vi "Configure Measurement (Spectrum Emission Mask).vi"(0 "VISA resource name":refnum<visa-resource-name>, 1 "Channel Span (2E+7 Hz)":dbl=20000000.0, 2 "Enable Averaging (T: Enable)":bool=TRUE, 5 "Auto Resolution Bandwidth (T: Enable)":bool=TRUE, 7 "Resolution Bandwidth (30 Hz)":dbl=30.0, 9 "Center Frequency (1E+9 Hz)":dbl=1000000000.0, 11 "error in (no error)":errorcluster, 12 "Average Number (20)":dbl=20.0) -> (4 "VISA resource name out":refnum<visa-resource-name>, 15 "error out":errorcluster)   [LabVIEW 2022 SP3, in "Agilent N934X Series.lvlib"]
doc: "Sets the Spectrum Emission Mask measurement parameters.\n\nNote:\nThis VI is only applicable for N9321C, N9322C, N9323C, N9324C models"
uses:
  <instrlib>/Agilent N934X Series/Agilent N934X Series.lvlib
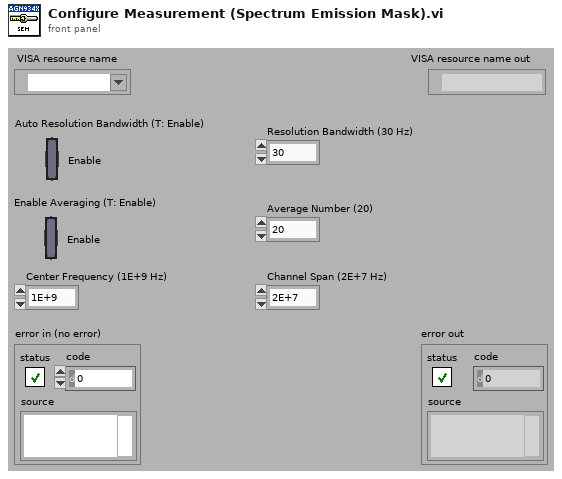
[diagram p1: front panel]
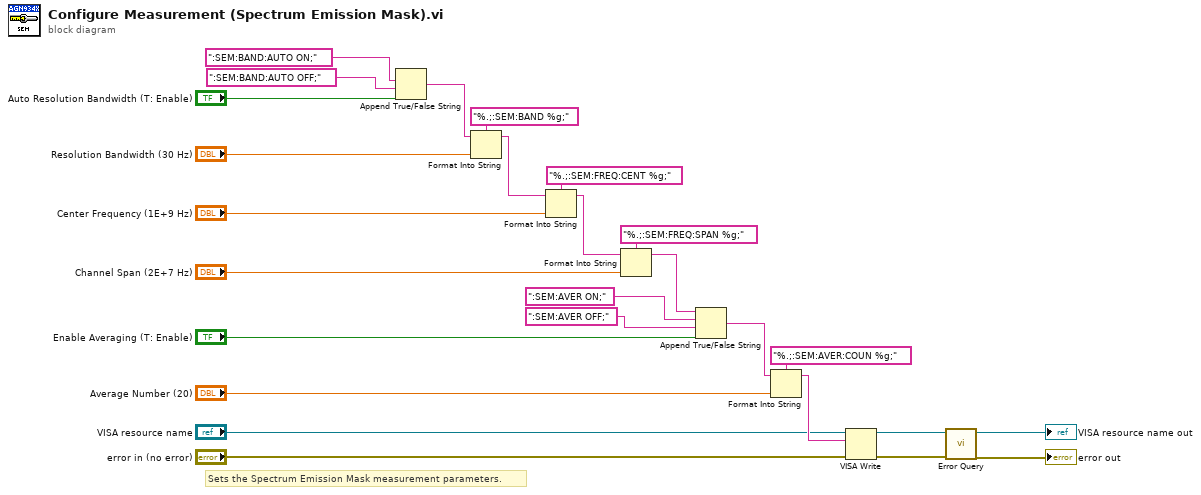
[diagram p0: block diagram]
diagram:
  # "Sets the Spectrum Emission Mask measurement parameters."
  n1 = Append True/False String(1:"Auto Resolution Bandwidth (T: Enable)", 2:":SEM:BAND:AUTO OFF;", 3:":SEM:BAND:AUTO ON;") -> (0:w23:string)  [unwired: 1 in]
  n2 = Format Into String(format string="%.;:SEM:BAND %g;", initial string=w23, "Resolution Bandwidth (30 Hz)") -> (resulting string=w20:string)  [unwired: 1 in, 1 out]
  n3 = Format Into String(format string="%.;:SEM:FREQ:CENT %g;", initial string=w20, "Center Frequency (1E+9 Hz)") -> (resulting string=w17:string)  [unwired: 1 in, 1 out]
  n4 = Format Into String(format string="%.;:SEM:FREQ:SPAN %g;", initial string=w17, "Channel Span (2E+7 Hz)") -> (resulting string=w14:string)  [unwired: 1 in, 1 out]
  n5 = Append True/False String(1:"Enable Averaging (T: Enable)", 2:":SEM:AVER OFF;", 3:":SEM:AVER ON;", 4:w14) -> (0:w10:string)
  n6 = Format Into String(format string="%.;:SEM:AVER:COUN %g;", initial string=w10, "Average Number (20)") -> (resulting string=w7:string)  [unwired: 1 in, 1 out]
  n7 = VISA Write(VISA resource name="VISA resource name", write buffer=w7, error in (no error)="error in (no error)") -> (VISA resource name out=w4:refnum<visa-resource-name>, error out=w3:errorcluster)  [unwired: 1 out]
  n8 = call <instrlib>:"Error Query.vi"("error in (no error)"=w3, "VISA resource name"=w4) -> ("error out"=→"error out":errorcluster, "VISA resource name out"=→"VISA resource name out":refnum<visa-resource-name>)  [unwired: 6 in, 2 out]
